vi "read_calibration_file.vi"(0 "configuration file path":path, 11 "error in (no error)":errorcluster) -> (4 "Calibration Data":cluster{"quad_term":dbl, "linear_term":dbl}, 15 "error out":errorcluster)   [LabVIEW 2023]
uses:
  <vilib>/Utility/config.llb/Read Key (Double).vi
  <vilib>/Utility/config.llb/NI_LVConfig.lvlib
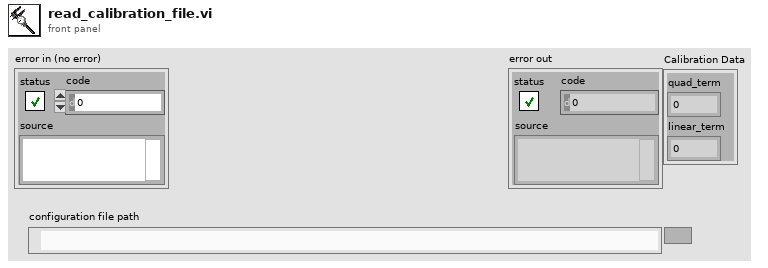
[diagram p1: front panel]
types:
  T1 = typedef "NI_LVConfig.lvlib/Config Data RefNum.ctl" = refnum<k1>
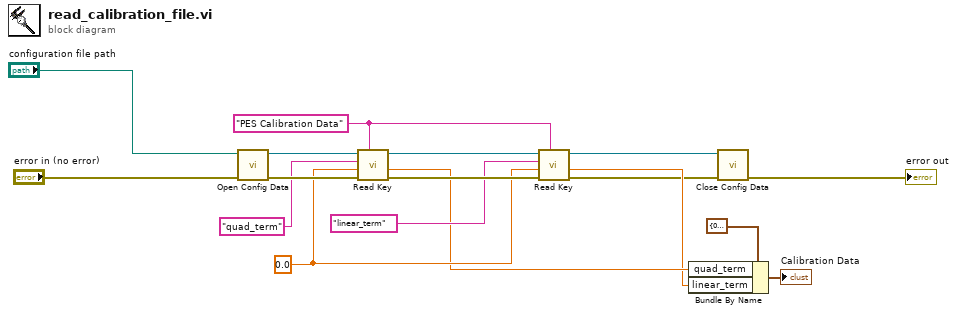
[diagram p0: block diagram]
diagram:
  w10 = 0.0
  w13 = "PES Calibration Data" ("section")
  n1 = call <vilib>:"Open Config Data.vi"("error in (no error)"="error in (no error)", "configuration file path"="configuration file path") -> ("error out"=w16:errorcluster, "refnum"=w17:T1)  [unwired: 7 in, 1 out]
  n2 = call-poly <vilib>:"Read Key.vi"("section"=w13, "error in (no error)"=w16, "default value"=w10, "key"="quad_term", "refnum"=w17) -> ("error out"=w14:errorcluster, "value"=w8:dbl, "refnum out"=w15:T1)  [unwired: 3 in, 1 out]
  n3 = call-poly <vilib>:"Read Key.vi"("section"=w13, "error in (no error)"=w14, "default value"=w10, "key"="linear_term", "refnum"=w15) -> ("error out"=w5:errorcluster, "value"=w7:dbl, "refnum out"=w6:T1)  [unwired: 3 in, 1 out]
  n4 = Bundle By Name(cluster=cluster{"quad_term":dbl, "linear_term":dbl} {"quad_term"=0.0, "linear_term"=0.0}, "quad_term"=w8, "linear_term"=w7) -> (→"Calibration Data":cluster{"quad_term":dbl, "linear_term":dbl})
  n5 = call <vilib>:"Close Config Data.vi"("error in (no error)"=w5, "refnum"=w6) -> ("error out"=→"error out":errorcluster)  [unwired: 8 in, 1 out]
